vi "rhozero_test.vi"(11 "Q in":dbl) -> (3 "rho0 value out":dbl)   [LabVIEW 2018]
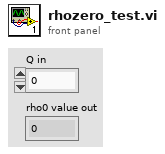
[diagram p1: front panel]
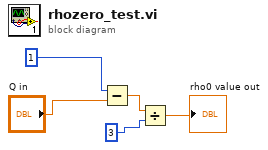
[diagram p0: block diagram]
diagram:
  n1 = Subtract(x=1, y="Q in") -> (x-y=w3:dbl)
  n2 = Divide(x=w3, y=3) -> (x/y=→"rho0 value out":dbl)
